vi "Handle Error.vi"(8 "error in (no error)":errorcluster, 11 "Controls in":refnum<class "Controls.lvclass">) -> (0 "error out":errorcluster, 2 "stop actor?":bool=TRUE, 3 "Controls out":refnum<class "Controls.lvclass">)   [LabVIEW 2020, in "Controls.lvlib" / "Controls.lvclass"]
doc: "(<B>Filename</B>: Actor Framework.lvlib:Actor.lvclass:Handle Error.vi)\n\nDefines how the actor handles an error that occurred while processing a message. By default, this method does nothing except stop the actor."
uses:
  Controls.lvclass
  <vilib>/ActorFramework/Actor/Actor.lvclass
  Controls.lvclass/Controls.ctl
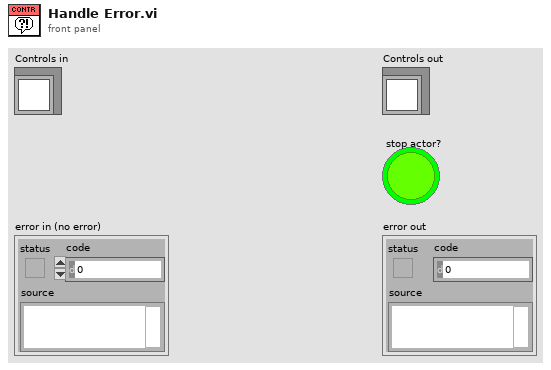
[diagram p1: front panel]
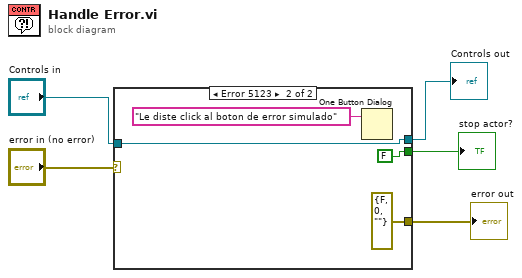
[diagram p0: block diagram]
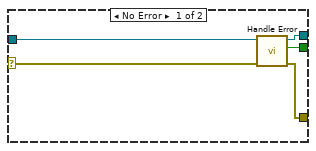
[diagram p2: hidden frame]
diagram:
  n1 = case shown="Error 5123" "error in (no error)" {
    selector: "error in (no error)" -> [w7 _]
    tunnel: [w10 errorcluster {"status"=FALSE, "code"=0, "source"=""} ("error out")] -> w5
    tunnel: [w9 FALSE ("stop actor?")] -> w4
    tunnel: [w8 w14] -> w3
    tunnel: "Controls in" -> [w6 w14]
    frame No Error {
      n2 = call-parent "Handle Error.vi"("error in (no error)"=w7, "Actor in"=w6) -> ("error out"=w10:errorcluster, "stop actor?"=w9:bool, "Actor out"=w8:refnum<class "Controls.lvclass">)  [unwired: 7 in]
    }
    frame Error {
      n3 = One Button Dialog(message="Le diste click al boton de error simulado") -> ()  [unwired: 1 in, 1 out]
    }
  }
  "Controls out" <- w3
  "error out" <- w5
  "stop actor?" <- w4
